vi "nanocal -- nuclear schottky fit V4.vi"() -> ()   [LabVIEW 2020] (continued)
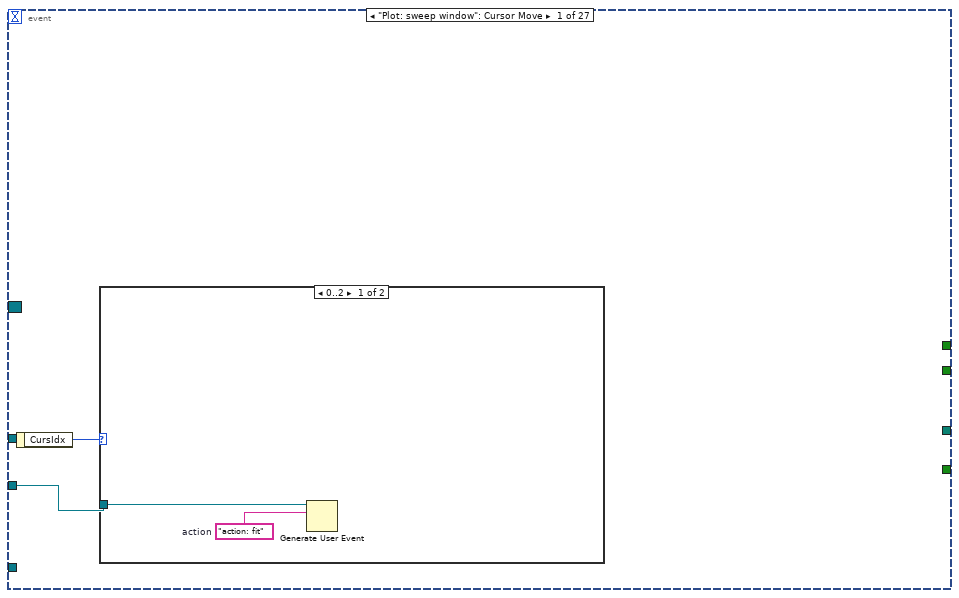
[diagram p2: hidden frame]
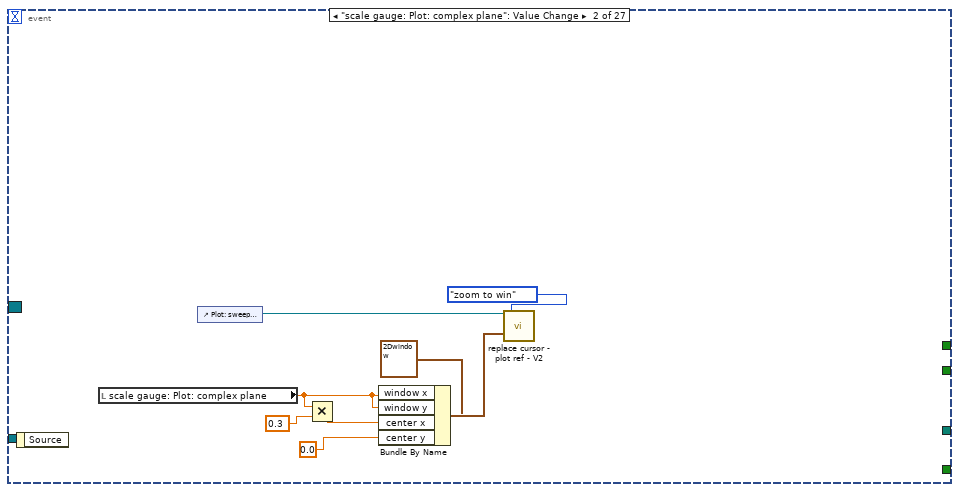
[diagram p4: hidden frame]
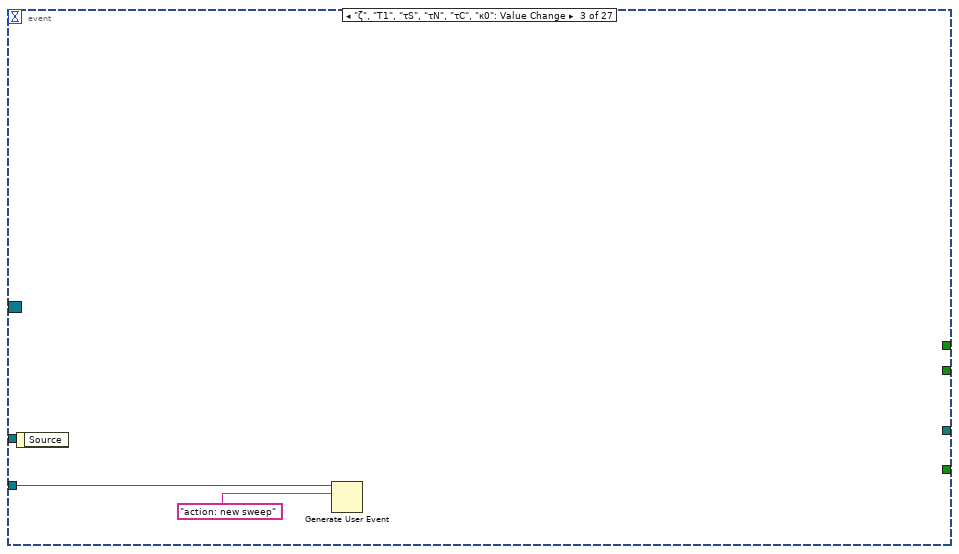
[diagram p5: hidden frame]
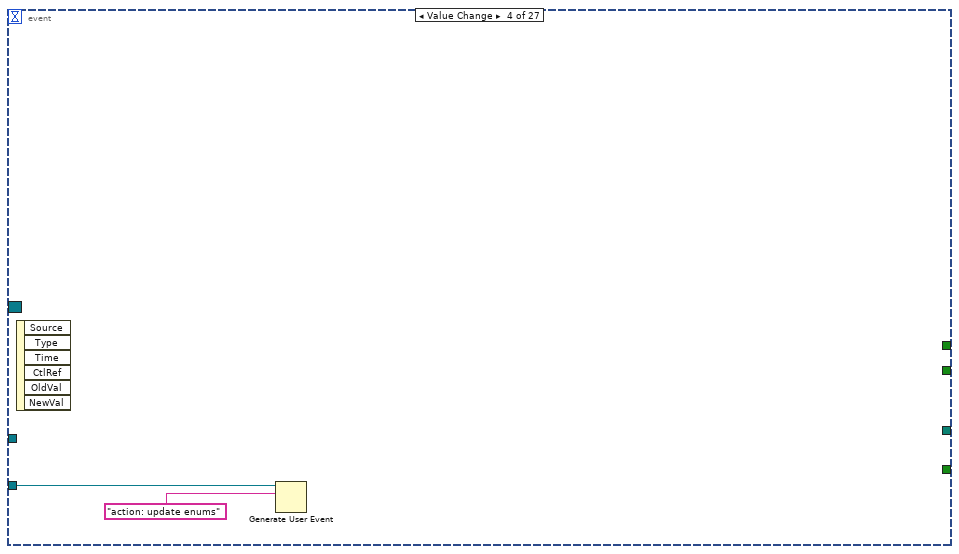
[diagram p6: hidden frame]
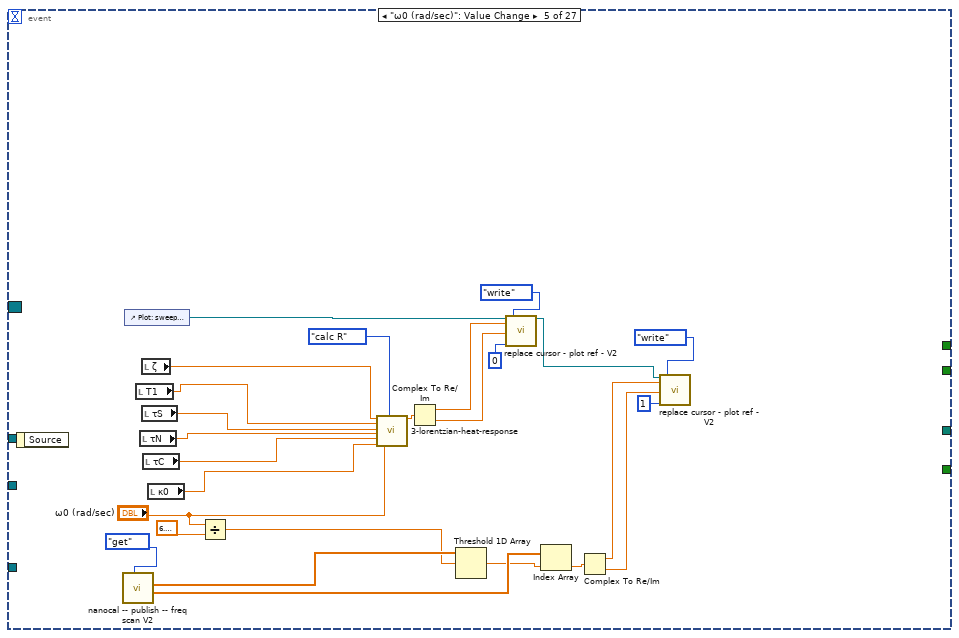
[diagram p7: hidden frame]
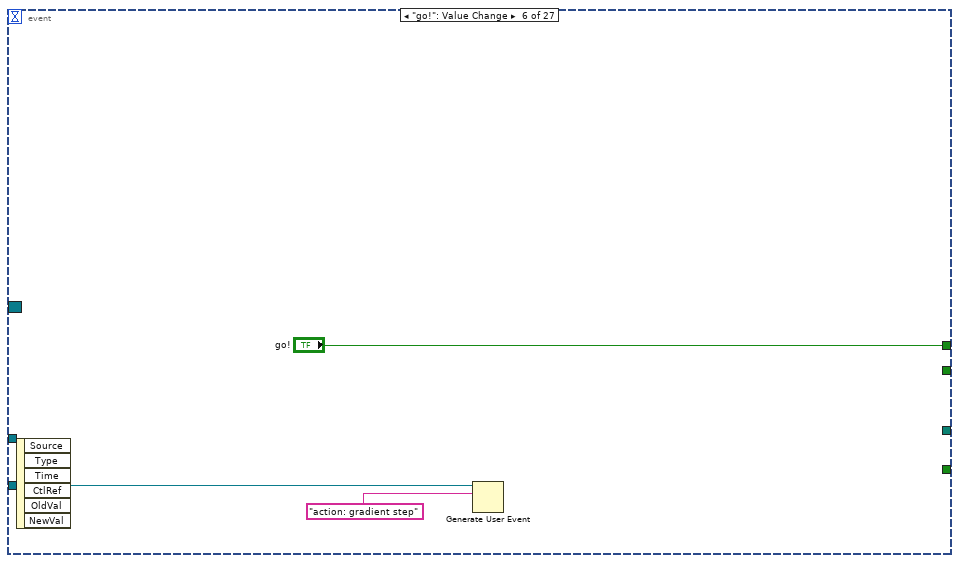
[diagram p8: hidden frame]
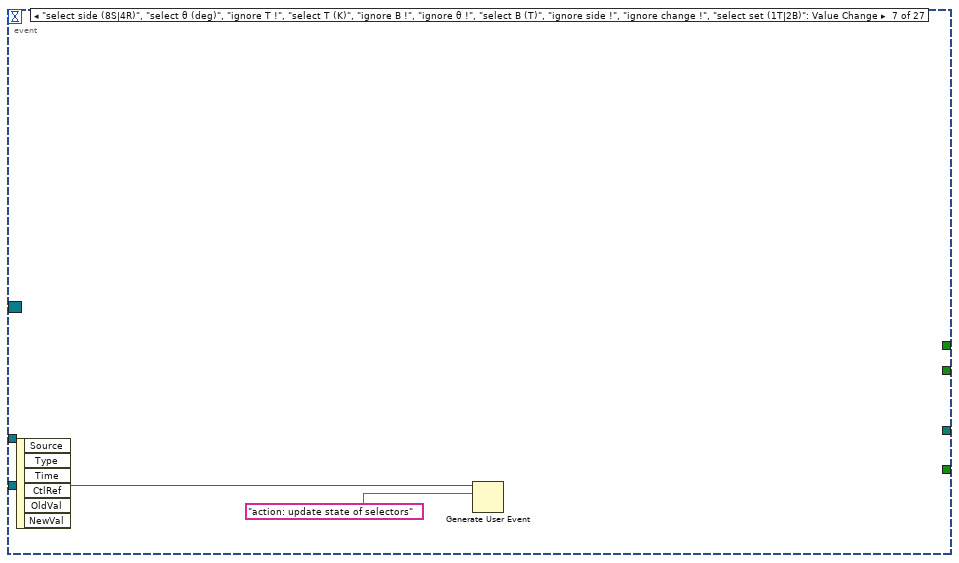
[diagram p9: hidden frame]
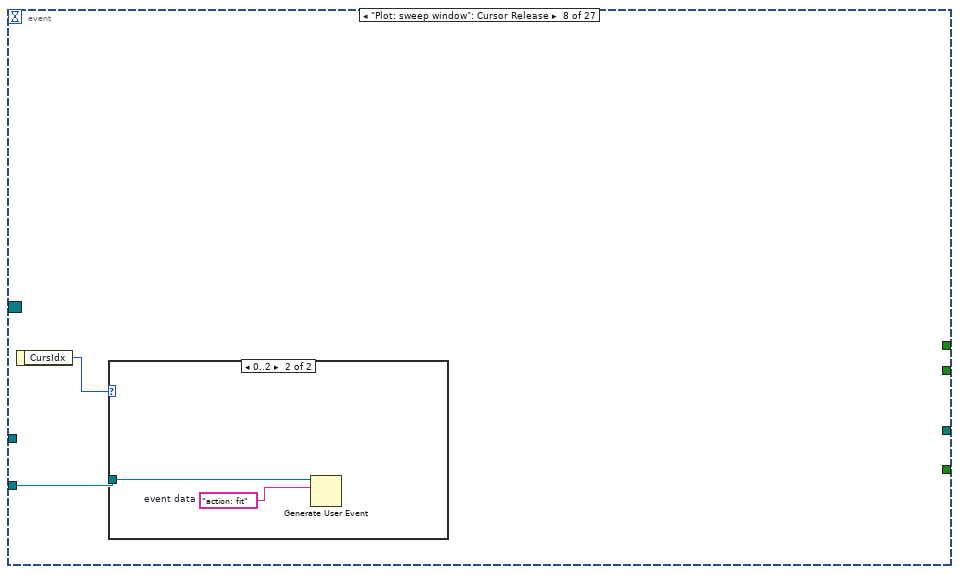
[diagram p10: hidden frame]
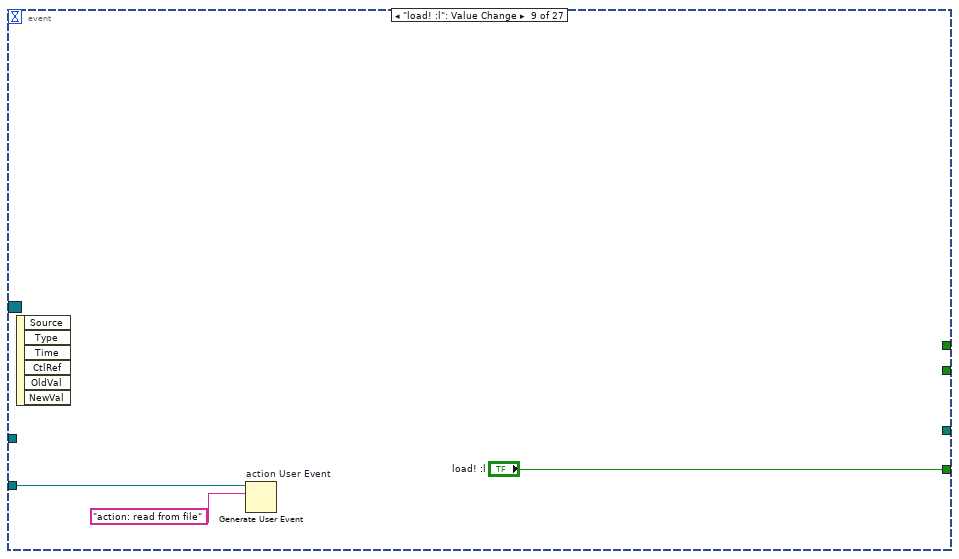
[diagram p12: hidden frame]
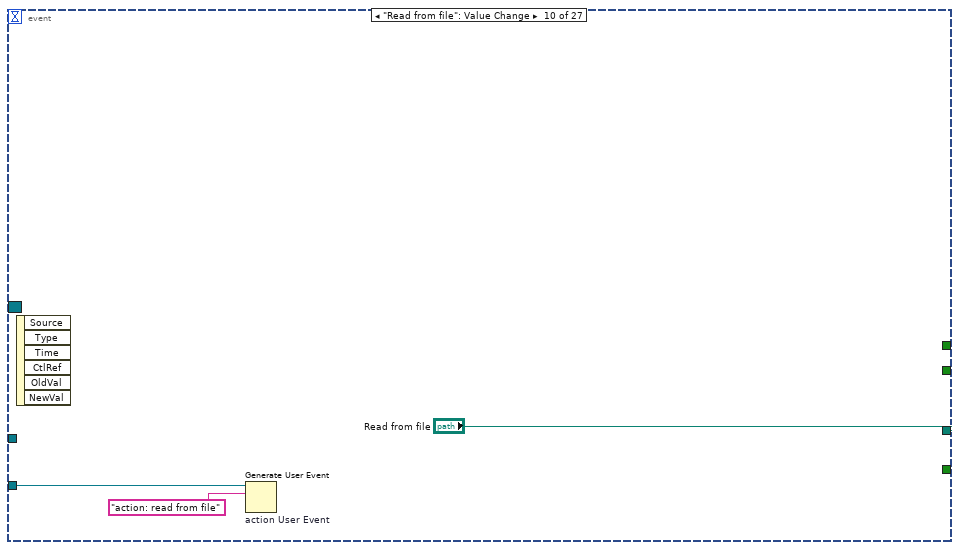
[diagram p13: hidden frame]
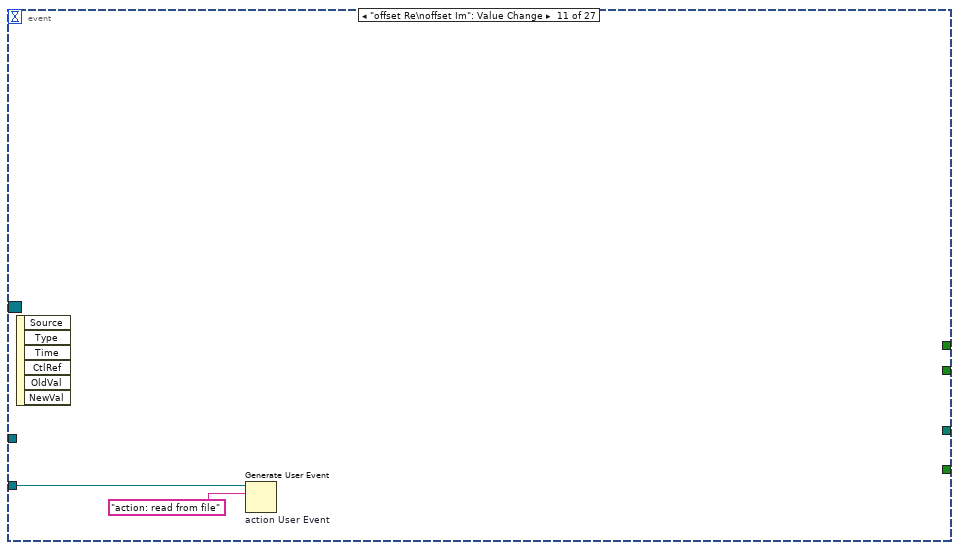
[diagram p14: hidden frame]
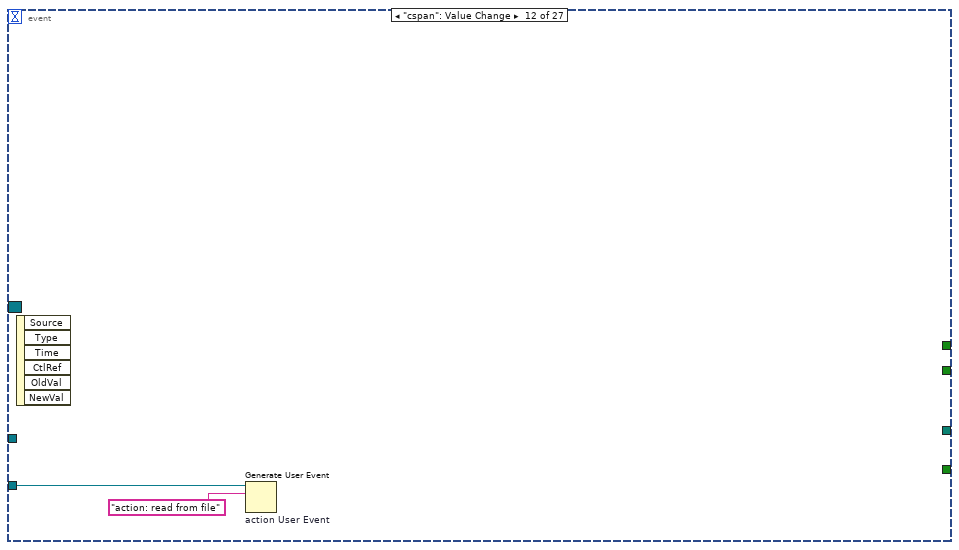
[diagram p15: hidden frame]
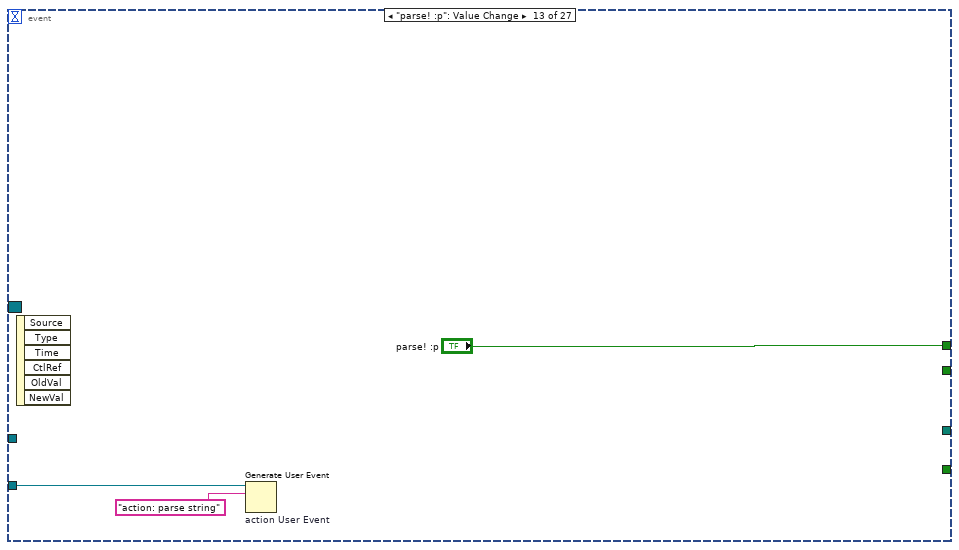
[diagram p16: hidden frame]
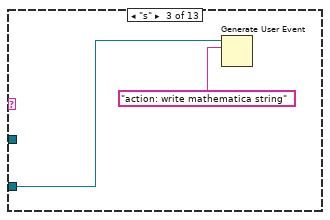
[diagram p19: hidden frame]
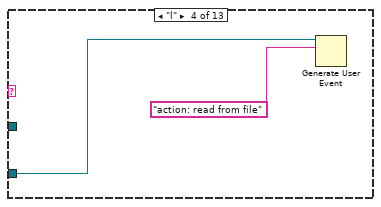
[diagram p20: hidden frame]
        n644 = event-data() -> ()  [unwired: 1 in, 6 out]
        n645 = Generate User Event "action User Event"(user event=w1245, event data cluster="action: read from file" ("event data")) -> ()  [unwired: 2 in, 2 out]
      }
      event "offset Re\noffset Im": Value Change {
        n646 = event-data() -> ()  [unwired: 1 in, 6 out]
        n647 = Generate User Event "action User Event"(user event=w1247, event data cluster="action: read from file" ("event data")) -> ()  [unwired: 2 in, 2 out]
      }
      event "cspan": Value Change {
        n648 = event-data() -> ()  [unwired: 1 in, 6 out]
        n649 = Generate User Event "action User Event"(user event=w1249, event data cluster="action: read from file" ("event data")) -> ()  [unwired: 2 in, 2 out]
      }
      event "parse! :p": Value Change {
        n650 = event-data() -> ()  [unwired: 1 in, 6 out]
        n651 = Generate User Event "action User Event"(user event=w1252, event data cluster="action: parse string" ("event data")) -> ()  [unwired: 2 in, 2 out]
      }
      event Key Down {
        n652 = event-data() -> ("Char"=w1256:i16, "VKey"=w1259:T31)  [unwired: 1 in]
        n653 = Build Array(w1256) -> (w1257:i16[])
        n654 = Byte Array To String(unsigned byte array=w1257) -> (string=w1255:string)
        n655 = case shown="\"ASCII\", Default" w1259 {
          selector: w1259 -> [_ _ _ _ _ _ w1317]
          tunnel: w1258 -> [w1262 _ _ w1312 _ _ _]
          tunnel: w1255 -> [w1261 _ _ _ _ _ _]
          tunnel: w1254 -> [w1260 _ _ _ _ _ w1316]
          frame "ASCII", Default {
            n656 = case shown="\"\\\\\", \"|\"" w1261 {
              selector: w1261 -> [_ _ _ _ _ _ w1274 _ _ _ _ w1290 _]
              tunnel: w1262 -> [_ _ w1263 w1265 w1268 _ _ _ w1281 w1284 w1286 w1288 w1309]
              tunnel: w1260 -> [_ _ _ _ _ w1272 _ _ _ _ _ _ _]
              frame "0", Default {
              }
              frame "a" {
              }
              frame "s" {
                n657 = Generate User Event(user event=w1263, event data cluster="action: write mathematica string" ("event data")) -> ()  [unwired: 2 in, 2 out]
              }
              frame "l" {
                n658 = Generate User Event(user event=w1265, event data cluster="action: read from file" ("event data")) -> ()  [unwired: 2 in, 2 out]
              }
              frame " " {
                n659 = Generate User Event(user event=w1268, event data cluster="action: gradient step" ("event data")) -> ()  [unwired: 2 in, 2 out]
              }
              frame "?" {
                # "?"
                n660 = call "replace cursor - plot ref - V2.vi"("Plot ref in"=w1272, "cursor action"=cursor_action."zoom to win") -> ("Plot ref out"=w1271:refnum<vi>)  [unwired: 14 in, 3 out]
                n661 = call "replace cursor - plot ref - V2.vi"("Plot ref in"=w1271, "cursor action"=cursor_action."smart zoom out&aspect") -> ()  [unwired: 14 in, 4 out]
              }
              frame "+", ",", "-", ".", "<", "=", ">" {
                n662 = local read "factor"() -> (w1276:dbl)
                n663 = case shown="\"0\", Default" w1274 {
                  tunnel: [0.7 1.0 1.5] -> w1273
                  frame ",", "-", "<" {
                  }
                  frame "0", Default {
                  }
                  frame "+", ".", "=", ">" {
                  }
                }
                n664 = Multiply(x=w1273, y=w1276) -> (x*y=w1275:dbl)
                n665 = local write "factor"(w1275) -> ()
              }
              frame "b" {
                n666 = local read "String"() -> (w1280:string)
                n667 = local write "backup string :b"(w1280) -> ()
              }
              frame "u" {
                n668 = Generate User Event(user event=w1281, event data cluster="ignoreaction: uco" ("event data")) -> ()  [unwired: 2 in, 2 out]
              }
              frame "p" {
                n669 = Generate User Event "action User Event"(user event=w1284, event data cluster="action: copy to math" ("event data")) -> ()  [unwired: 2 in, 2 out]
              }
              frame "q" {
                n670 = Generate User Event "action User Event"(user event=w1286, event data cluster="action: copy from math" ("event data")) -> ()  [unwired: 2 in, 2 out]
              }
              frame "\\", "|" {
                n671 = for {
                  N: 1 -> [_]
                  tunnel: w1290 -> [w1304]
                  tunnel: w1288 -> [w1303]
                  tunnel: [w1303] -> w1287
                  n672 = local read "constrained filenames :|\\"() -> (w1295:u16)
                  n673 = To Long Integer(number=w1295) -> (32bit integer=w1294:i32)
                  n674 = property on="constrained filenames :|\\" class="Ring (strict)"() -> ("NumItems"=w1293:u32)  [unwired: 2 in, 2 out]
                  n675 = case shown="\"|\", Default" w1304 {
                    tunnel: w1294 -> [w1306 w1308]
                    tunnel: [w1305 w1307] -> w1300
                    frame "|", Default {
                      n676 = Decrement(x=w1306) -> (x-1=w1305:i32)
                    }
                    frame "\\" {
                      n677 = Increment(x=w1308) -> (x+1=w1307:i32)
                    }
                  }
                  n678 = To Long Integer(number=w1293) -> (32bit integer=w1292:i32)
                  n679 = Greater Or Equal?(x=w1300, y=w1292) -> (x >= y?=w1302:bool)
                  n680 = Select(t=u16 0 ("lower limit"), s=w1302, f=w1300) -> (s? t:f=w1297:i32)
                  n681 = Decrement(x=w1292) -> (x-1=w1298:i32)
                  n682 = Less Than 0?(x=w1297) -> (x < 0?=w1299:bool)
                  n683 = Select(t=w1298, s=w1299, f=w1297) -> (s? t:f=w1296:i32)
                  n684 = local write "constrained filenames :|\\"(w1296) -> ()
                }
                n685 = Generate User Event ("action User Event")(user event=w1287, event data cluster="action: constrained filenames select" ("event data")) -> ()  [unwired: 2 in, 2 out]
              }
              frame "m" {
                n686 = Generate User Event "action User Event"(user event=w1309, event data cluster="action: copy from math" ("event data")) -> ()  [unwired: 2 in, 2 out]
              }
            }
          }
          frame "Escape" {
            n687 = local write "newton pause"(TRUE ("newton pause")) -> ()
          }
          frame "PageUp" {
          }
          frame "Enter" {
            n688 = Generate User Event ("action User Event")(user event=w1312, event data cluster="action: new sweep" ("event data")) -> (user event out=w1313:refnum<user-event>)  [unwired: 2 in, 1 out]
            n689 = Generate User Event ("action User Event")(user event=w1313, event data cluster="action: replot colors" ("event data")) -> ()  [unwired: 2 in, 2 out]
          }
          frame "Caps" {
          }
          frame "PageDown" {
          }
          frame "Up".."Right" {
            n690 = case shown="\"Down\"" w1317 {
              tunnel: [cursor_action."zoom in 20%" ("cursor action") cursor_action."zoom out 20%" ("cursor action") cursor_action."zoom out 20%" ("cursor action") cursor_action."zoom in 20%" ("cursor action")] -> w1318
              frame "Up", Default {
              }
              frame "Down" {
              }
              frame "Left" {
              }
              frame "Right" {
              }
            }
            n691 = call "replace cursor - plot ref - V2.vi"("Plot ref in"=w1316, "cursor action"=w1318) -> ()  [unwired: 14 in, 4 out]
          }
        }
      }
      event "Plot:  colors": Cursor Move {
        n692 = event-data() -> ("CursIdx"=w1326:i32)  [unwired: 1 in]
        n693 = local read "T1"() -> (w1342:dbl)
        n694 = local read "τS"() -> (w1343:dbl)
        n695 = local read "τN"() -> (w1344:dbl)
        n696 = local read "τC"() -> (w1345:dbl)
        n697 = local read "κ0"() -> (w1346:dbl)
        n698 = local read "ζ"() -> (w1341:dbl)
        n699 = call "replace cursor - plot ref - V2.vi"("Plot ref in"=w1347, "cursor index"=w1326, "cursor action"=cursor_action."read") -> ("read Y"=w1325:dbl)  [unwired: 13 in, 3 out]
        n700 = Build Array(w1341, w1342, w1343, w1344, w1345, w1346) -> (w1328:dbl[])
        n701 = Replace Array Subset(array=w1328, new element=w1325, index=w1326) -> (w1327:dbl[])
        n702 = Generate User Event(user event=w1324, event data cluster="action: replot circles" ("event data")) -> ()  [unwired: 2 in, 2 out]
        n703 = Index Array(array=w1327, index #1=0 ("index"), index #2=1 ("index"), index #3=2 ("index"), index #4=3 ("index"), index #5=4 ("index"), index #6=5 ("index")) -> (element #1=w1334:dbl, element #2=w1333:dbl, element #3=w1332:dbl, element #4=w1331:dbl, element #5=w1330:dbl, element #6=w1329:dbl)
        n704 = local write "τN"(w1331) -> ()
        n705 = local write "τC"(w1330) -> ()
        n706 = local write "τS"(w1332) -> ()
        n707 = local write "κ0"(w1329) -> ()
        n708 = local write "T1"(w1333) -> ()
        n709 = local write "ζ"(w1334) -> ()
      }
      event "pause!": Value Change {
        n710 = event-data() -> ()  [unwired: 1 in, 6 out]
        n711 = local write "newton pause"(TRUE ("newton pause")) -> ()
      }
      event "uco! :u": Value Change {
        n712 = event-data() -> ()  [unwired: 1 in, 1 out]
        n713 = Generate User Event(user event=w1352, event data cluster="ignoreaction: uco" ("event data")) -> ()  [unwired: 2 in, 2 out]
      }
      event "read τ from Math ! :q": Value Change {
        n714 = event-data() -> ()  [unwired: 1 in, 1 out]
        n715 = Generate User Event(user event=w1355, event data cluster="action: copy from math" ("event data")) -> ()  [unwired: 2 in, 2 out]
      }
      event "write τ to Math! :p": Value Change {
        n716 = event-data() -> ()  [unwired: 1 in, 1 out]
        n717 = Generate User Event(user event=w1358, event data cluster="action: copy to math" ("event data")) -> ()  [unwired: 2 in, 2 out]
      }
      event "Math --> string OUT  ! :s": Value Change {
        n718 = event-data() -> ()  [unwired: 1 in, 1 out]
        n719 = Generate User Event(user event=w1361, event data cluster="action: write mathematica string" ("event data")) -> ()  [unwired: 2 in, 2 out]
      }
      event "generate empty string from filelist !": Value Change {
        n720 = event-data() -> ()  [unwired: 1 in, 1 out]
        n721 = Generate User Event(user event=w1364, event data cluster="action: empty string from filelist" ("event data")) -> ()  [unwired: 2 in, 2 out]
      }
      event "string IN  --> Math!": Value Change {
        n722 = event-data() -> ()  [unwired: 1 in, 1 out]
        n723 = Generate User Event(user event=w1367, event data cluster="action: read mathematica string" ("event data")) -> ()  [unwired: 2 in, 2 out]
      }
      event "filenames": Value Change {
        n724 = event-data() -> ()  [unwired: 1 in, 6 out]
        n725 = local read "filesnames lookup"() -> (w1374:map{i32, string})
        n726 = local read "all full filenames"() -> (w1372:map{string, path})
        n727 = local read "filenames"() -> (w1373:u16)
        n728 = Look In Map(map=w1374, key=w1373) -> (value=w1371:string)  [unwired: 1 in, 1 out]
        n729 = Look In Map(map=w1372, key=w1371) -> (value=w1369:path)  [unwired: 1 in, 1 out]
        n730 = for {
          N: 1 -> [_]
          tunnel: w1375 -> [w1377]
          tunnel: w1369 -> [w1376]
          n731 = local write "Read from file"(w1376) -> ()
          n732 = Generate User Event(user event=w1377, event data cluster="action: read from file" ("event data")) -> ()  [unwired: 2 in, 2 out]
        }
      }
      event "constrained filenames :|\\": Value Change {
        n733 = event-data() -> ()  [unwired: 1 in, 6 out]
        n734 = Generate User Event(user event=w1379, event data cluster="action: constrained filenames select" ("event data")) -> ()  [unwired: 2 in, 2 out]
      }
      event User Event {
        n735 = event-data() -> ("interface"=w1382:string)  [unwired: 1 in, 4 out]
        n736 = case shown="\"interface: update color cursors\"" w1382 {
          tunnel: [_ _ TRUE] -> w1381
          frame "void", Default {
          }
          frame "interface: update color cursors" {
            w1386 = T5[] [enum."T (K)", enum."B (T)", enum."θ (deg)"] items=["ζ", "τ1", "τS", "τN", "τC", "κ0", "m1", "m2", "m3", "T (K)", "B (T)", "θ (deg)", "side (S|R)", "change (B|T)"]
            w1383 = T5[] [enum."ζ", enum."τ1", enum."τS", enum."τN", enum."τC", enum."κ0", enum."m1", enum."m2", enum."m3"] items=["ζ", "τ1", "τS", "τN", "τC", "κ0", "m1", "m2", "m3", "T (K)", "B (T)", "θ (deg)", "side (S|R)", "change (B|T)"]
            n737 = local read "T1"() -> (w1394:dbl)
            n738 = local read "τS"() -> (w1395:dbl)
            n739 = local read "τN"() -> (w1396:dbl)
            n740 = local read "τC"() -> (w1397:dbl)
            n741 = local read "κ0"() -> (w1398:dbl)
            n742 = local read "ζ"() -> (w1393:dbl)
            n743 = local read "cursor x selector"() -> (w1389:map{T5, dbl})
            n744 = local read "X selector"() -> (w1390:T5)
            n745 = local read "T (K)"() -> (w1391:dbl)
            n746 = Build Array(w1393, w1394, w1395, w1396, w1397, w1398) -> (w1400:dbl[])
            n747 = Look In Map(map=w1389, key=w1390, default value=w1391) -> (value=w1392:dbl)  [unwired: 1 out]
            n748 = local read "θ (deg)"() -> (w1404:dbl)
            n749 = local read "B (T)"() -> (w1403:dbl)
            n750 = local read "T (K)"() -> (w1402:dbl)
            n751 = for {
              shift-right: [w1416] -> w1401
              shift-left: map{T5, dbl} {} ("Map IN") -> [w1417]
              tunnel: w1383 -> [w1414] mode=indexing
              tunnel: w1400 -> [w1415] mode=indexing
              tunnel: [w1414] -> w1409 mode=indexing
              n752 = Insert Into Map(map in=w1417, key=w1414, value=w1415) -> (map out=w1416:map{T5, dbl})  [unwired: 2 out]
            }
            n753 = control-ref of="Plot:  colors"() -> (w1388:refnum<vi>)
            n754 = local read "cursor index map"() -> (w1399:map{T5, i32})
            n755 = Build Array(w1402, w1403, w1404) -> (w1406:dbl[])
            n756 = call "3-lorentzian-heat-response -- V4.vi"("action"=3-lorentzian-heat-response_action."calc m1m2m3", "Map IN"=w1401) -> ("Map OUT"=w1405:map{T5, dbl})  [unwired: 7 in, 2 out]
            n757 = for {
              shift-right: [w1412] -> w1407
              shift-left: w1405 -> [w1413]
              tunnel: w1386 -> [w1411] mode=indexing
              tunnel: w1406 -> [w1410] mode=indexing
              n758 = Insert Into Map(map in=w1413, key=w1411, value=w1410) -> (map out=w1412:map{T5, dbl})  [unwired: 2 out]
            }
            n759 = for {
              tunnel: w1392 -> [w1425]
              tunnel: w1388 -> [w1424]
              tunnel: w1409 -> [w1420] mode=indexing
              tunnel: w1399 -> [w1422]
              shift-right: [w1419] -> _
              shift-left: w1405 -> [w1419]
              n760 = Look In Map(map=w1419, key=w1420) -> (value=w1418:dbl)  [unwired: 1 in, 1 out]
              n761 = Look In Map(map=w1422, key=w1420) -> (value=w1421:i32)  [unwired: 1 in, 1 out]
              n762 = call "replace cursor - plot ref - V2.vi"("Plot ref in"=w1424, "new X"=w1425, "new  Y"=w1418, "cursor index"=w1421, "cursor action"=cursor_action."write") -> ()  [unwired: 11 in, 4 out]
            }
            n763 = call "string parse mathematica assosiated array.vi"("derivative"=mathematica_string_map_action."create string", "Map IN"=w1407) -> ("String OUT"=w1408:string)  [unwired: 8 in, 1 out]
            n764 = local write "String"(w1408) -> ()
          }
          frame "interface: exit" {
          }
        }
      }
      event "plot landscape!", "range one", "range two": Value Change {
        n765 = event-data() -> ()  [unwired: 1 in, 6 out]
        n766 = Generate User Event(user event=w1427, event data cluster="action: plot landscape" ("event data")) -> ()  [unwired: 2 in, 2 out]
      }
      event "colors": Value Change {
        n767 = event-data() -> ()  [unwired: 1 in, 6 out]
        n768 = Generate User Event(user event=w1430, event data cluster="action: reset colors" ("event data")) -> ()  [unwired: 2 in, 2 out]
      }
    }
  }
  "cursor x selector" <- w36
